vi "Fetch Measurement (Channel Power).vi"(8 "error in (no error)":errorcluster, 9 "Timeout (20000 ms)":i32=20000, 11 "VISA resource name":refnum<visa-resource-name>) -> (0 "error out":errorcluster, 1 "Power Spectral Density":dbl format="%#.6g", 2 "Channel Power":dbl format="%#.6g", 3 "VISA resource name out":refnum<visa-resource-name>)   [LabVIEW 2014, in "Agilent ESA PSA Series.lvlib"]
doc: "Returns the results of the last measurement(Channel Power) and does not initiate data acquisition."
uses:
  Agilent ESA PSA Series.lvlib
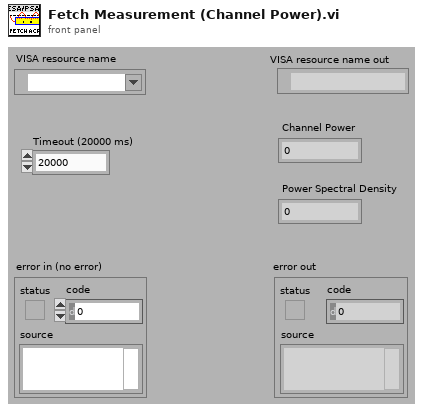
[diagram p1: front panel]
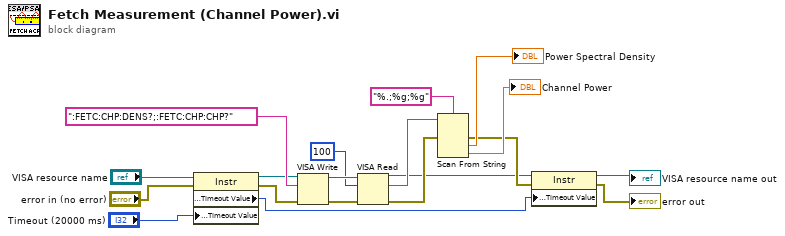
[diagram p0: block diagram]
diagram:
  n1 = property on="Property Node" class="Instr"(reference="VISA resource name", error in="error in (no error)", "General Settings:Timeout Value"="Timeout (20000 ms)") -> (reference out=w8:refnum<visa-resource-name>, error out=w7:errorcluster, "General Settings:Timeout Value"=w2:u32)
  n2 = VISA Write(VISA resource name=w8, write buffer=":FETC:CHP:DENS?;:FETC:CHP:CHP?" ("format string"), error in (no error)=w7) -> (VISA resource name out=w18:refnum<visa-resource-name>, error out=w19:errorcluster)  [unwired: 1 out]
  n3 = VISA Read(VISA resource name=w18, byte count=u32 100, error in (no error)=w19) -> (VISA resource name out=w3:refnum<visa-resource-name>, read buffer=w15:string, error out=w16:errorcluster)  [unwired: 1 out]
  n4 = Scan From String(format string="%.;%g;%g", input string=w15, error in=w16) -> (error out=w4:errorcluster, output 1=→"Power Spectral Density":dbl, output 2=→"Channel Power":dbl)  [unwired: 3 in, 2 out]
  n5 = property on="Property Node" class="Instr"(reference=w3, error in=w4, "General Settings:Timeout Value"=w2) -> (reference out=→"VISA resource name out":refnum<visa-resource-name>, error out=→"error out":errorcluster)
